vi "HexDecode.vi"(10 "Input":string) -> (0 "Width":dbl, 1 "Y":dbl, 2 "X":dbl, 3 "Color":dbl, 4 "Height":dbl)   [LabVIEW 2016]
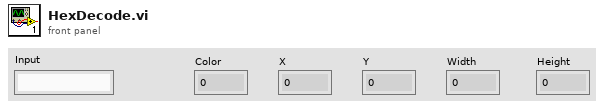
[diagram p1: front panel]
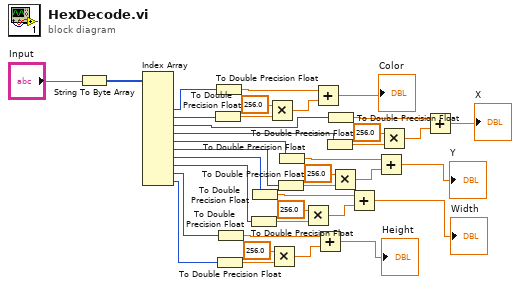
[diagram p0: block diagram]
diagram:
  n1 = String To Byte Array(string="Input") -> (unsigned byte array=w36:u8[])
  n2 = Index Array(array=w36) -> (element #3=w35:u8, element #4=w34:u8, element #5=w25:u8, element #6=w24:u8, element #7=w20:u8, element #8=w19:u8, element #9=w13:u8, element #10=w12:u8, element #11=w8:u8, element #12=w6:u8)  [unwired: 12 in, 2 out]
  n3 = To Double Precision Float(number=w34) -> (double precision float=w33:dbl)
  n4 = To Double Precision Float(number=w35) -> (double precision float=w30:dbl)
  n5 = To Double Precision Float(number=w6) -> (double precision float=w7:dbl)
  n6 = To Double Precision Float(number=w8) -> (double precision float=w9:dbl)
  n7 = To Double Precision Float(number=w12) -> (double precision float=w17:dbl)
  n8 = To Double Precision Float(number=w13) -> (double precision float=w14:dbl)
  n9 = Multiply(x=256.0, y=w33) -> (x*y=w31:dbl)
  n10 = Multiply(x=256.0, y=w7) -> (x*y=w10:dbl)
  n11 = To Double Precision Float(number=w19) -> (double precision float=w18:dbl)
  n12 = To Double Precision Float(number=w20) -> (double precision float=w21:dbl)
  n13 = Multiply(x=256.0, y=w17) -> (x*y=w15:dbl)
  n14 = Add(x=w30, y=w31) -> (x+y=→"Color":dbl)
  n15 = Add(x=w9, y=w10) -> (x+y=→"Height":dbl)
  n16 = To Double Precision Float(number=w24) -> (double precision float=w29:dbl)
  n17 = To Double Precision Float(number=w25) -> (double precision float=w26:dbl)
  n18 = Multiply(x=256.0, y=w18) -> (x*y=w22:dbl)
  n19 = Add(x=w14, y=w15) -> (x+y=→"Width":dbl)
  n20 = Add(x=w21, y=w22) -> (x+y=→"Y":dbl)
  n21 = Multiply(x=256.0, y=w29) -> (x*y=w27:dbl)
  n22 = Add(x=w26, y=w27) -> (x+y=→"X":dbl)
